vi "Read Parameters Dirty.vi"(8 "error in (no error)":errorcluster, 11 "VoiceMeeterRemote in":refnum<class "VoiceMeeterRemote.lvclass">) -> (0 "error out":errorcluster, 2 "Parameters Dirty?":bool, 3 "VoiceMeeterRemote out":refnum<class "VoiceMeeterRemote.lvclass">)   [LabVIEW 2022 SP3, in "VoiceMeeterRemote.lvlib" / "VoiceMeeterRemote.lvclass"]
uses:
  VoiceMeeterRemote.lvclass
  VoiceMeeterRemote.lvclass/VoiceMeeterRemote.ctl
  VoiceMeeterRemote.lvlib
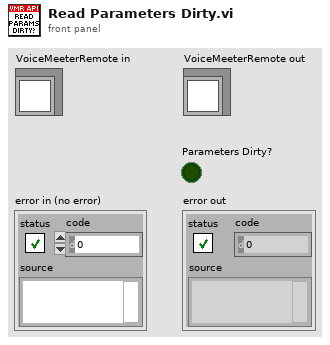
[diagram p1: front panel]
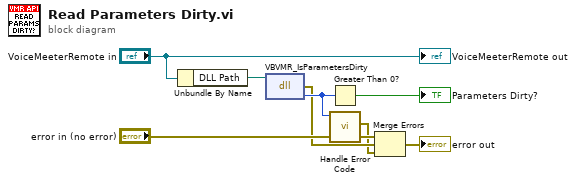
[diagram p0: block diagram]
diagram:
  n1 = Unbundle By Name("VoiceMeeterRemote in") -> ("DLL Path"=w6:path)
  n2 = dll-call lib="C:/Program Files/National Instruments/LabVIEW 2022/user.lib/VoicemeeterRemote64/VoicemeeterRemote64.*" fn="VBVMR_IsParametersDirty"(path in=w6) -> (error out=w2:errorcluster, "return type"=w4:i32)  [unwired: 2 in, 1 out]
  n3 = Greater Than 0?(x=w4) -> (x > 0?=→"Parameters Dirty?":bool)
  n4 = call "Handle Error Code.vi"("Code"=w4) -> ("error out"=w1:errorcluster)  [unwired: 10 in]
  n5 = Merge Errors("error in (no error)", w2, w1) -> (→"error out":errorcluster)
  "VoiceMeeterRemote out" <- "VoiceMeeterRemote in"
